vi "SRV_VAR.vi"(0 "SuperPro in":T1, 1 "Name":string, 2 "type":T2(ring)=enum."i8") -> (3 "SuperPro out":T1, 4 "Name":string, 5 "type out":T2(ring), 6 "Variables":T3(array[cluster]))   [LabVIEW 2009]
uses:
  <userlib>/SuperPro/OpCodes/_SubVIs/SuperProControl.ctl
panel:
  out "new":bool
  # "This LabVIEW item is deprecated.\n\nIt is believed to be unused and will be removed in a future version of SRV."
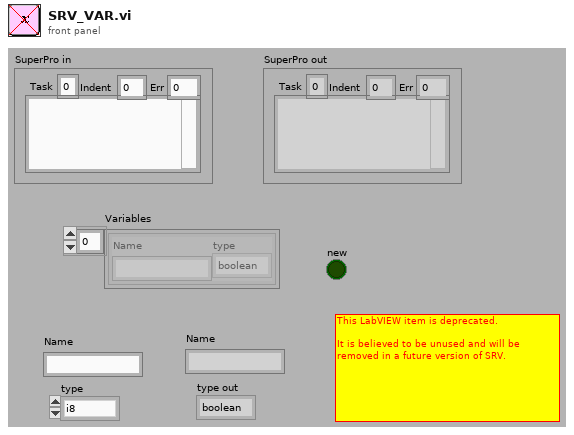
[diagram p1: front panel]
types:
  T1 = typedef "SuperProControl.ctl" = cluster{"Task":i32, "Indent":i32, "Err":i32, "ASM":string}
  T2 = enum16{"boolean", "u8", "i8", "u16", "i16", "u32", "i32", "u64", "i64", "SGL", "DBL", "EXT", "CPX"}
  T3 = cluster{"Name":string, "type":enum16{"boolean", "u8", "i8", "u16", "i16", "u32", "i32", "u64", "i64", "SGL", "DBL", "EXT", "CPX"}}[]
  T4 = cluster{"Name":string, "type":enum16{"boolean", "u8", "i8", "u16", "i16", "u32", "i32", "u64", "i64", "SGL", "DBL", "EXT", "CPX"}}
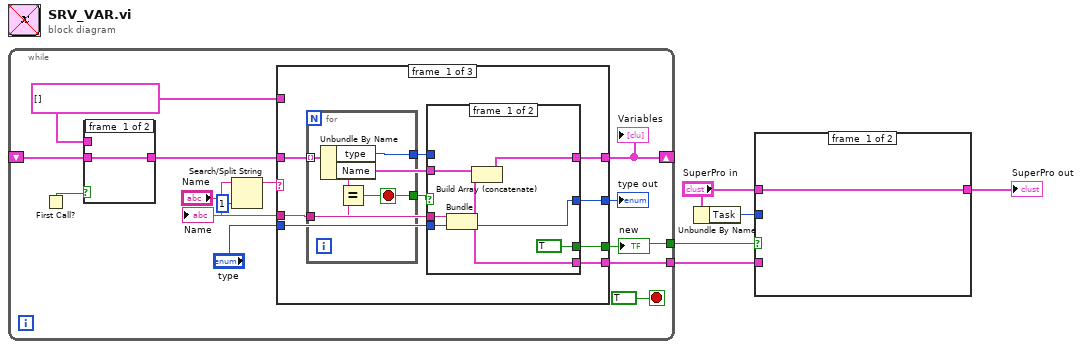
[diagram p0: block diagram]
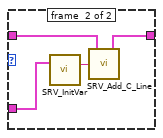
[diagram p3: hidden frame]
diagram:
  n1 = while {
    shift-right: [w18] -> _
    shift-left: _ -> [w10]
    tunnel: [w7] -> w5
    tunnel: [w6] -> w3
    stop <- TRUE stop-if-true
    w9 = T3 [] ("Variables")
    n2 = First Call?() -> (First Call?: T/F=w12:bool)
    n3 = case shown="False" w12 {
      tunnel: [w19 w20] -> w11
      tunnel: w10 -> [w19 _]
      tunnel: w9 -> [_ w20]
      frame #0 {
      }
      frame #1 {
      }
    }
    n4 = Search/Split String(string="Name", offset (0)=1) -> (substring before match=w14:string)  [unwired: 1 in, 2 out]
    n5 = case shown="Default" w14 {
      tunnel: [w26 w44 w46] -> w18
      tunnel: w11 -> [w28 w44 _]
      tunnel: "type" -> [w27 w43 w45]
      tunnel: "Name" -> [w25 _ _]
      tunnel: w9 -> [_ _ w46]
      tunnel: [w24 w43 w45] -> w8
      tunnel: [w22 _ _] -> w7
      tunnel: [w21 _ _] -> w6
      frame #0 {
        n6 = for {
          tunnel: w28 -> [w42] mode=indexing
          tunnel: w25 -> [w41]
          tunnel: [w39] -> w29
          tunnel: [w38] -> w23
          stop <- w39 stop-if-true
          n7 = Unbundle By Name(w42) -> ("type"=w38:T2, "Name"=w40:string)
          n8 = Equal?(x=w40, y=w41) -> (x = y?=w39:bool)
        }
        n9 = case shown="True" w29 {
          tunnel: w28 -> [w35 w37]
          tunnel: w25 -> [w34 _]
          tunnel: w27 -> [w32 _]
          tunnel: [w33 w37] -> w26
          tunnel: [w32 w36] -> w24
          tunnel: w23 -> [_ w36]
          tunnel: [TRUE _] -> w22
          tunnel: [w30 _] -> w21
          frame #0 {
            n10 = Bundle("Name"=w34, "type"=w32) -> (w30:T4)  [unwired: 1 in]
            n11 = Build Array (concatenate)(w35, w30) -> (w33:T3)
          }
          frame #1 {
          }
        }
      }
      frame #1 {
      }
      frame #2 {
      }
    }
    "Variables" <- w18
    "type out" <- w8
    "new" <- w7
    "Name" <- "Name"
  }
  n12 = Unbundle By Name("SuperPro in") -> ("Task"=w1:i32)
  n13 = case shown="True" w5 {
    tunnel: "SuperPro in" -> [w47 w51]
    tunnel: [w47 w50] -> w4
    tunnel: w3 -> [_ w49]
    tunnel: w1 -> [_ w48]
    frame #0 {
    }
    frame #1 {
      n14 = case shown="-1" w48 {
        tunnel: w51 -> [w52 w56]
        tunnel: [w52 w55] -> w50
        tunnel: w49 -> [_ w54]
        frame #0 {
        }
        frame #1 {
          n15 = call "SRV_InitVar.vi"("Variable"=w54) -> ("String"=w53:string)  [unwired: 1 in]
          n16 = call "SRV_Add_C_Line.vi"("C String"=w53, "SuperPro in"=w56) -> ("SuperPro out"=w55:T1)  [unwired: 3 in]
        }
      }
    }
  }
  "SuperPro out" <- w4
